vi "CRYUpdate Curve Library Graph.vi"(5 "sOption 2":string, 7 "sOption 1":string="Some", 8 "Deleted Names":string[](array[string]), 9 "Replaced Old Names":string[](array[string]), 10 "Index":i32[](array[numeric]), 11 "Type":enum16{"Curves", "Values", "Results", "WFM"}(ring)) -> ()   [LabVIEW 2013]
uses:
  CRYWindow/SubVI/CRYMain Sub Window Global.vi
panel:
  # "Unprotect All Data(Curves, Values,Results, Waveforms)"
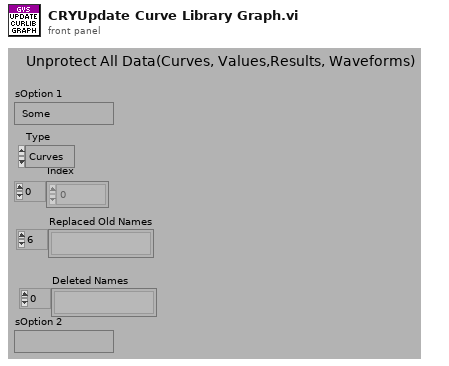
[diagram p1: front panel]
types:
  T1 = typedef "CRYResult Cluster Array.ctl" = T2[]
  T2 = typedef "CRYResult Cluster.ctl" = cluster{"Name":string, "Margin":dbl, "unit":string, "Verdict":bool, "Limit":string, "Max/Min":string, "protected":bool, "Step No.":i32, "Test Info":string, "AutoProtect":bool}
  T3 = typedef "CRYData Cluster Array.ctl" = T4[]
  T4 = typedef "CRYData Cluster.ctl" = cluster{"Name":string, "Curve":cluster{"x":dbl, "y":dbl, "z":dbl}[], "X data":u16, "Y data":u16, "Z data":u16, "X axis":u16, "Y axis":u16, "Z axis":u16, "X unit":string, "Y unit":string, "Z unit":string, "X dB ref":dbl, "Y dB ref":dbl, "Z dB ref":dbl, "single val":bool, "protected":bool, "display X":bool, "display Y":bool, "display Z":bool, "Test Info":string, "Step No.":i32, "Plot Settings":cluster{"Color":u32, "Interpolation":u8, "Point Style":u8, "Line Style":u8, "Point Color":u32, "Line Width":u8, "Bar Plot Style":u8, "Fill To":i16}, "AutoProtect":bool}
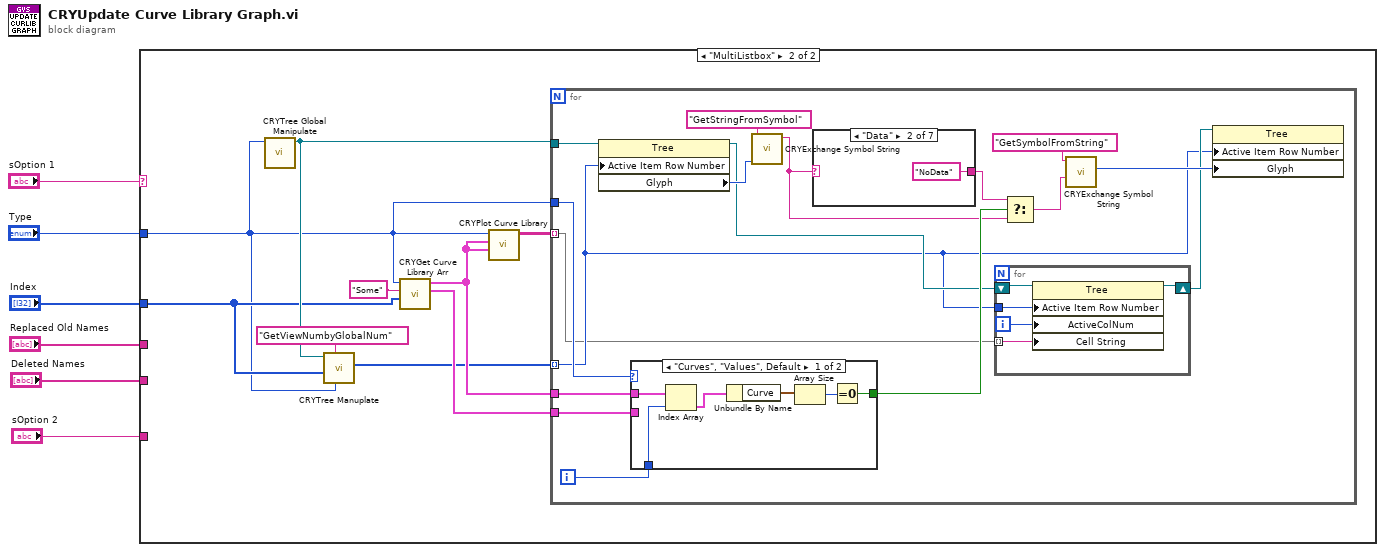
[diagram p0: block diagram]
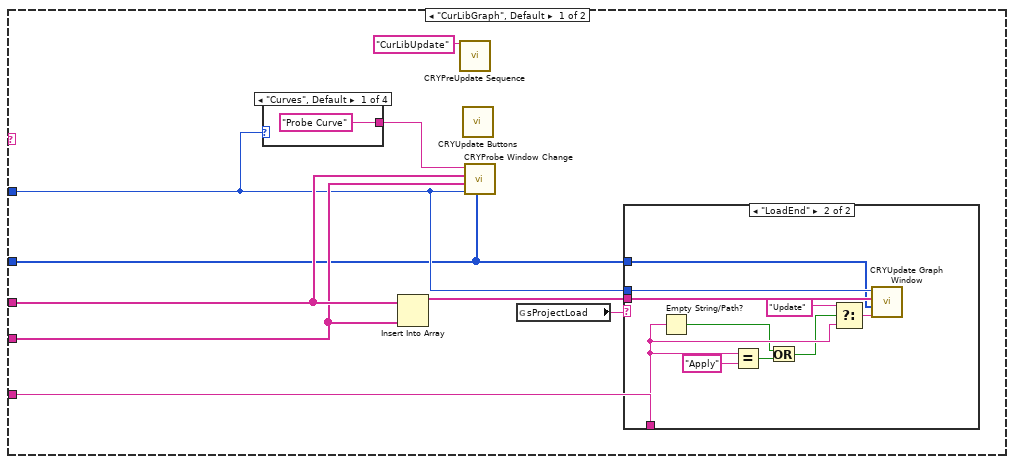
[diagram p2: hidden frame]
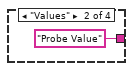
[diagram p4: hidden frame]
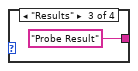
[diagram p5: hidden frame]
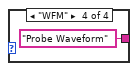
[diagram p6: hidden frame]
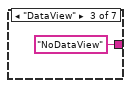
[diagram p8: hidden frame]
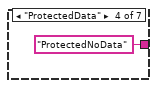
[diagram p9: hidden frame]
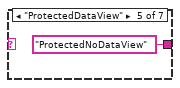
[diagram p10: hidden frame]
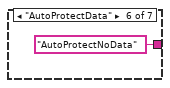
[diagram p11: hidden frame]
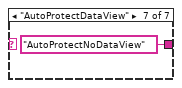
[diagram p12: hidden frame]
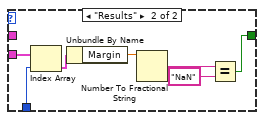
[diagram p13: hidden frame]
diagram:
  n1 = case shown="\"MultiListbox\"" "sOption 1" {
    tunnel: "Index" -> [w7 w32]
    tunnel: "Type" -> [w11 w30]
    tunnel: "Replaced Old Names" -> [w13 _]
    tunnel: "Deleted Names" -> [w12 _]
    tunnel: "sOption 2" -> [w8 _]
    frame "CurLibGraph", Default {
      n2 = case shown="\"Curves\", Default" w11 {
        tunnel: ["Probe Curve" "Probe Value" "Probe Result" "Probe Waveform"] -> w10
        frame "Curves", Default {
        }
        frame "Values" {
        }
        frame "Results" {
        }
        frame "WFM" {
        }
      }
      n3 = Insert Into Array(array=w13, new element=w12) -> (w15:string[])  [unwired: 1 in]
      n4 = call "CRYPreUpdate Sequence.vi"("EventName"="CurLibUpdate") -> ()  [unwired: 15 in]
      n5 = call "CRYUpdate Buttons.vi"() -> ()  [unwired: 1 in, 11 out]
      n6 = call "CRYProbe Window Change.vi"("Update Index"=w7, "Type"=w11, "Close Names"=w12, "Update Names"=w13, "Probe Type"=w10) -> ()  [unwired: 7 out]
      n7 = global read "CRYMain Sub Window Global.vi" "sProjectLoad"() -> (w9:string)
      n8 = case shown="\"LoadEnd\"" w9 {
        tunnel: w15 -> [_ w25]
        tunnel: w11 -> [_ w24]
        tunnel: w8 -> [_ w20]
        tunnel: w7 -> [_ w21]
        frame Default {
        }
        frame "LoadEnd" {
          n9 = Empty String/Path?(string/path=w20) -> (empty?=w17:bool)
          n10 = Equal?(x=w20, y="Apply") -> (x = y?=w18:bool)
          n11 = Or(x=w17, y=w18) -> (x .or. y?=w16:bool)
          n12 = Select(t="Update" ("sOption"), s=w16, f=w20) -> (s? t:f=w23:string)
          n13 = call "CRYUpdate Graph Window.vi"("sOption"=w23, "Index"=w21, "Del/Update Names"=w25, "Type"=w24) -> ()  [unwired: 1 in, 7 out]
        }
      }
    }
    frame "MultiListbox" {
      n14 = call "CRYTree Global Manipulate.vi"("Type In"=w30) -> ("Tree/Curve Tree"=w33:refnum<vi>)  [unwired: 7 in, 3 out]
      n15 = call "CRYTree Manuplate.vi"("Type"=w30, "sAction"="GetViewNumbyGlobalNum", "nData"=w32, "Tree in"=w33) -> ("nData Out"=w31:i32[])  [unwired: 4 in, 3 out]
      n16 = call "CRYGet Curve Library Arr.vi"("Index"=w32, "sOption"="Some", "Type In"=w30) -> ("Results"=w36:T1, "Curves/Values"=w35:T3)  [unwired: 6 in, 1 out]
      n17 = call "CRYPlot Curve Library.vi"("Values"=w35, "Curves"=w35, "Type"=w30) -> ("PlotStrings"=w38:string[][])  [unwired: 8 in]
      n18 = for {
        tunnel: w38 -> [w39] mode=indexing
        tunnel: w33 -> [w47]
        tunnel: w31 -> [w40] mode=indexing
        tunnel: w36 -> [w53]
        tunnel: w35 -> [w55]
        tunnel: w30 -> [w54]
        i -> [w52]
        n19 = property on="Property Node" class="Tree"(reference=w47, "Active Item Row Number"=w40) -> (reference out=w42:refnum<vi>, "Glyph"=w50:i32)  [unwired: 1 in, 1 out]
        n20 = case shown="\"Curves\", \"Values\", Default" w54 {
          tunnel: w55 -> [w70 _]
          tunnel: [w71 w78] -> w46
          tunnel: w53 -> [_ w76]
          tunnel: w52 -> [w68 w74]
          frame "Curves", "Values", Default {
            n21 = Index Array(array=w70, index=w68) -> (element=w69:T4)
            n22 = Unbundle By Name(w69) -> ("Curve"=w73:cluster{"x":dbl, "y":dbl, "z":dbl}[])
            n23 = Array Size(array=w73) -> (size(s)=w72:i32)
            n24 = Equal To 0?(x=w72) -> (x = 0?=w71:bool)
          }
          frame "Results" {
            n25 = Index Array(array=w76, index=w74) -> (element=w75:T2)
            n26 = Unbundle By Name(w75) -> ("Margin"=w80:dbl)
            n27 = Number To Fractional String(number=w80) -> (F-format string=w79:string)  [unwired: 3 in]
            n28 = Equal?(x=w79, y="NaN") -> (x = y?=w78:bool)
          }
        }
        n29 = call "CRYExchange Symbol String.vi"("nData"=w50, "sAction"="GetStringFromSymbol") -> ("sData out"=w43:string)  [unwired: 8 in, 1 out]
        n30 = case shown="\"Data\"" w43 {
          selector: w43 -> [w56 _ _ _ _ _ _]
          tunnel: [w56 "NoData" ("sAction") "NoDataView" ("sAction") "ProtectedNoData" ("sAction") "ProtectedNoDataView" ("sAction") "AutoProtectNoData" ("sAction") "AutoProtectNoDataView" ("sAction")] -> w44
          frame Default {
          }
          frame "Data" {
          }
          frame "DataView" {
          }
          frame "ProtectedData" {
          }
          frame "ProtectedDataView" {
          }
          frame "AutoProtectData" {
          }
          frame "AutoProtectDataView" {
          }
        }
        n31 = for {
          shift-right: [w66] -> w41
          shift-left: w42 -> [w67]
          tunnel: w40 -> [w65]
          tunnel: w39 -> [w63] mode=indexing
          i -> [w64]
          n32 = property on="Property Node" class="Tree"(reference=w67, "Active Item Row Number"=w65, "ActiveColNum"=w64, "Cell String"=w63) -> (reference out=w66:refnum<vi>)  [unwired: 1 in, 1 out]
        }
        n33 = Select(t=w44, s=w46, f=w43) -> (s? t:f=w45:string)
        n34 = call "CRYExchange Symbol String.vi"("sData"=w45, "sAction"="GetSymbolFromString") -> ("nData out"=w48:i32)  [unwired: 8 in, 1 out]
        n35 = property on="Property Node" class="Tree"(reference=w41, "Active Item Row Number"=w40, "Glyph"=w48) -> ()  [unwired: 1 in, 2 out]
      }
    }
  }
